vi "CCD_ROI.vi"(0 "Raw Image":T2(plugin-control)=refnum caption="Raw image", 2 "Angle (degrees)":sgl(slide) scale=0.0..360.0, 3 "Type of Symmetry":u32(ring)=5 items=["Horizontal", "Vertical", "Central", "1st Diagonal", "2nd Diagonal", "No change"], 5 "Rectangle":T1, 6 "Image Logging Path":path, 7 "Log Image":bool) -> (14 "Transformed image":T2(plugin-control))   [LabVIEW 2016]
uses:
  <vilib>/vision/NI_Vision_Development_Module.lvlib
panel:
  in  "Overlay Thickness":i32(slide)=1 min=0 max=20 step=1 scale=0.0..20.0
  in  "error out 2":errorcluster
  out "error out":errorcluster
  in  "Color Palette":cluster{"Red":u8, "Green":u8, "Blue":u8}[](array[cluster])
  out "Rect image":T2(plugin-control)
  in  "Drawing Mode (Frame)":u32(ring) items=["Frame", "Fill", "Highlight"]
  in  "Color":u32(colorbox)=16711680
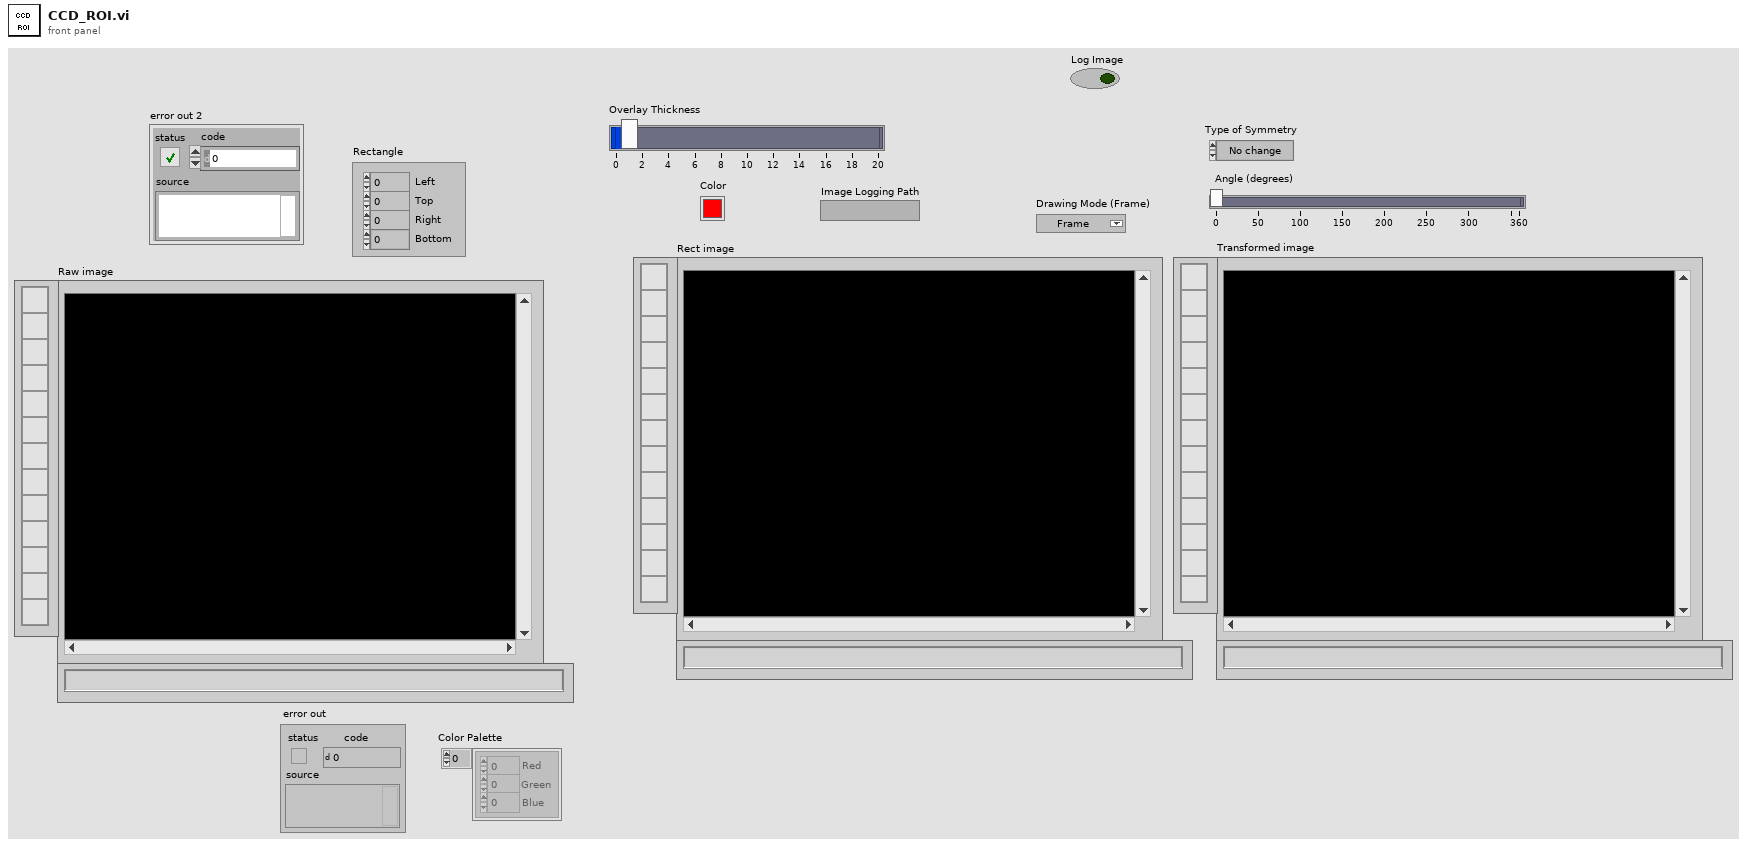
[diagram p1: front panel]
types:
  T1 = cluster{"Left":i32, "Top":i32, "Right":i32, "Bottom":i32}
  T2 = typedef "IMAQ Image.ctl" = refnum<image>
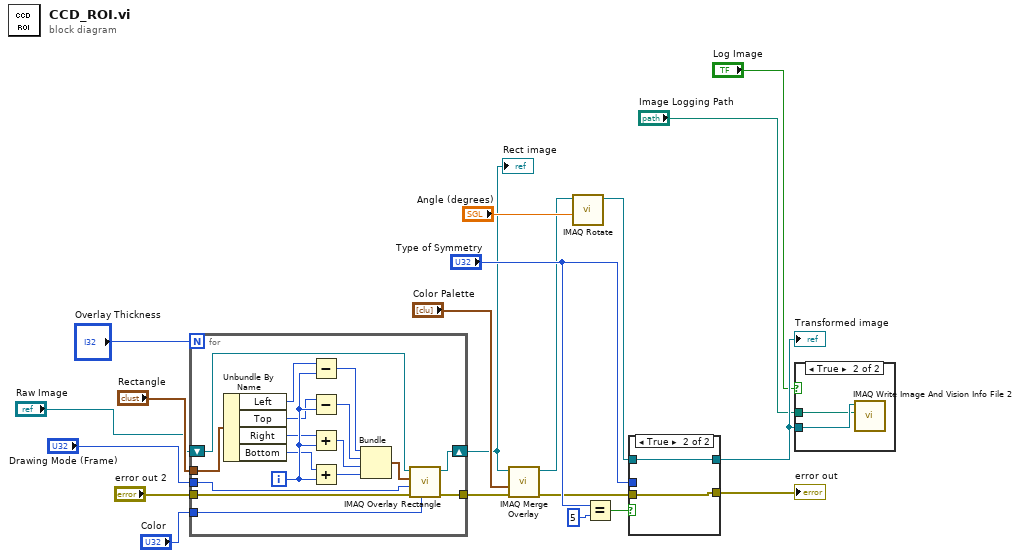
[diagram p0: block diagram]
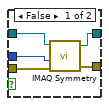
[diagram p3: hidden frame]
diagram:
  n1 = for {
    N: "Overlay Thickness" -> [_]
    tunnel: "Color" -> [w37]
    tunnel: "Drawing Mode (Frame)" -> [w33]
    tunnel: "Rectangle" -> [w30]
    tunnel: [w36] -> w2
    shift-right: [w34] -> w3
    shift-left: "Raw Image" -> [w35]
    tunnel: "error out 2" -> [w21]
    i -> [w32]
    n2 = Unbundle By Name(w30) -> ("Left"=w31:i32, "Top"=w28:i32, "Right"=w29:i32, "Bottom"=w27:i32)
    n3 = Subtract(x=w31, y=w32) -> (x-y=w26:i32)
    n4 = Subtract(x=w28, y=w32) -> (x-y=w25:i32)
    n5 = Add(x=w29, y=w32) -> (x+y=w24:i32)
    n6 = Add(x=w27, y=w32) -> (x+y=w23:i32)
    n7 = Bundle(w26, w25, w24, w23) -> (w22:cluster{i32, i32, i32, i32})  [unwired: 1 in]
    n8 = call "IMAQ Overlay Rectangle"("Color"=w37, "error in (no error)"=w21, "Drawing Mode (Frame)"=w33, "Rectangle"=w22, "Image"=w35) -> ("error out"=w36:errorcluster, "Image Out"=w34:T2)  [unwired: 5 in]
  }
  "Rect image" <- w3
  n9 = call "IMAQ Merge Overlay"("error in (no error)"=w2, "Color Palette"="Color Palette", "Image Src"=w3) -> ("error out"=w13:errorcluster, "Image Dst Out"=w14:T2)  [unwired: 7 in]
  n10 = call "IMAQ Rotate"("Angle (degrees)"="Angle (degrees)", "Image Src"=w14) -> ("Image Dst Out"=w19:T2)  [unwired: 8 in, 1 out]
  n11 = Equal?(x="Type of Symmetry", y=u32 5) -> (x = y?=w16:bool)
  n12 = case shown="True" w16 {
    tunnel: "Type of Symmetry" -> [w42 _]
    tunnel: w19 -> [w41 w44]
    tunnel: [w40 w44] -> w11
    tunnel: w13 -> [w39 w43]
    tunnel: [w38 w43] -> w12
    frame False {
      n13 = call "IMAQ Symmetry"("error in (no error)"=w39, "Type of Symmetry"=w42, "Image Src"=w41) -> ("error out"=w38:errorcluster, "Image Dst Out"=w40:T2)  [unwired: 2 in]
    }
    frame True {
    }
  }
  "Transformed image" <- w11
  "error out" <- w12
  n14 = case shown="True" "Log Image" {
    tunnel: w11 -> [_ w46]
    tunnel: "Image Logging Path" -> [_ w45]
    frame False {
    }
    frame True {
      n15 = call "IMAQ Write Image And Vision Info File 2"("File Path"=w45, "Image"=w46) -> ()  [unwired: 8 in, 2 out]
    }
  }
